vi "Source and Measure Current in DMM - Copy.vi"() -> ()   [LabVIEW 2021]
uses:
  NIDCpower/NIDCPower T12.lvlib
  NIDMM/Meas T12.ctl
  NIDCpower/controls/Config.ctl
  NIDMM/LoadDMM t12.ctl
panel:
  in  "Name 2":T1
  out "Name":T1
  in  "Load SMU":T2={"Range (Amps)"=0.2, "Resolution in Digits"=5.5} {"Resolution in Digits" items=["3 1/2"=3.5, "4 1/2"=4.5, "5 1/2"=5.5, "6 1/2"=6.5, "7 1/2"=7.5]; "Range (Amps)" format="%.2p"}
  in  "Cluster":T3={"Current Level"=0.01, "Current Level Range"=0.01, "Voltage Limit"=2.0, "Voltage Limit Range"=6.0, "Source Delay (Sec)"=0.1} {"Source Delay (Sec)" format="%.3p"; "Voltage Limit Range" format="%.5p"; "Voltage Limit" format="%.5p"; "Current Level Range" format="%.3p"; "Current Level" format="%.3p"}
  in  "Load DMM":refnum<k15>="Dev1"
  in  "error in":errorcluster
  out "error out":errorcluster
  in  "Load SMU Channel":string="0"
  in  "Load SMU":refnum<k15>="Dev1"
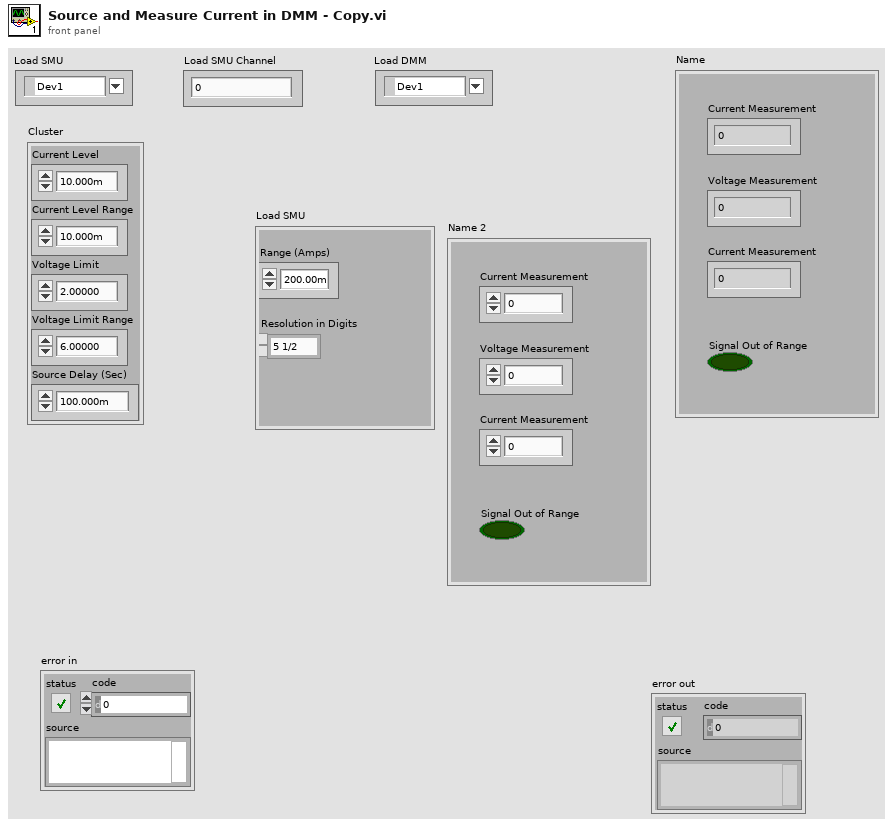
[diagram p1: front panel]
types:
  T1 = typedef "Meas T12.ctl" = cluster{"Current Measurement":dbl, "Voltage Measurement":dbl, "Signal Out of Range":bool, "Current in DMM":dbl}
  T2 = typedef "LoadDMM t12.ctl" = cluster{"Range (Amps)":dbl, "Resolution in Digits":dbl}
  T3 = typedef "NIDCPower T12.lvlib/Config.ctl" = cluster{"Current Level":dbl, "Current Level Range":dbl, "Voltage Limit":dbl, "Voltage Limit Range":dbl, "Source Delay (Sec)":dbl}
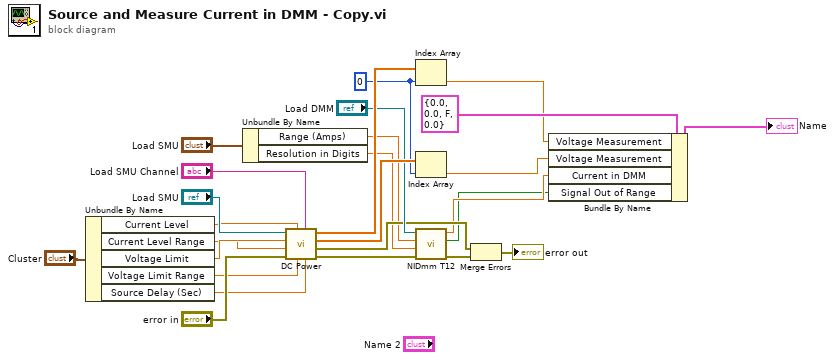
[diagram p0: block diagram]
diagram:
  w24 = 0 ("index")
  n1 = Unbundle By Name("Cluster") -> ("Current Level"=w14:dbl, "Current Level Range"=w12:dbl, "Voltage Limit"=w13:dbl, "Voltage Limit Range"=w11:dbl, "Source Delay (Sec)"=w10:dbl)
  n2 = Unbundle By Name("Load SMU") -> ("Range (Amps)"=w8:dbl, "Resolution in Digits"=w7:dbl)
  n3 = call "DC Power.vi"("Source Delay (Sec)"=w10, "Load SMU Channel"="Load SMU Channel", "Voltage Limit Range"=w11, "Current Level"=w14, "error in (no error)"="error in", "Current Level Range"=w12, "Voltage Limit"=w13, "IVI Refnum in"="Load SMU") -> (0:"error out"=w18:errorcluster, 1:"error out"=w17:errorcluster, "current measurements"=w25:dbl[], "voltage measurements"=w26:dbl[])
  n4 = Index Array(array=w26, index=w24) -> (element=w4:dbl)
  n5 = Index Array(array=w25, index=w24) -> (element=w3:dbl)
  n6 = call "NIDmm T12.vi"("error in (no error)"=w18, "Range (Amps)"=w7, "Resolution in Digits"=w8, "IVI Refnum in"="Load DMM") -> ("error out"=w16:errorcluster, "Over Range?"=w1:bool, "Measurement"=w2:dbl)  [unwired: 5 in]
  n7 = Merge Errors(w17, w16) -> (→"error out":errorcluster)
  n8 = Bundle By Name(cluster=T1 {"Current Measurement"=0.0, "Voltage Measurement"=0.0, "Signal Out of Range"=FALSE, "Current in DMM"=0.0} ("Name"), "Voltage Measurement"=w4, "Voltage Measurement"=w3, "Current in DMM"=w2, "Signal Out of Range"=w1) -> (→"Name":T1)
